vi "Withdrawal $50.vi"(8 "error in (no error)":errorcluster, 11 "ATM Controller in":refnum<class "ATM Controller.lvclass">) -> (0 "error out":errorcluster, 3 "ATM Controller out":refnum<class "ATM Controller.lvclass">)   [LabVIEW 2019, in "ATM Controller.lvlib" / "ATM Controller.lvclass"]
uses:
  ATM Controller.lvclass
  ATM Controller.lvclass/ATM Controller.ctl
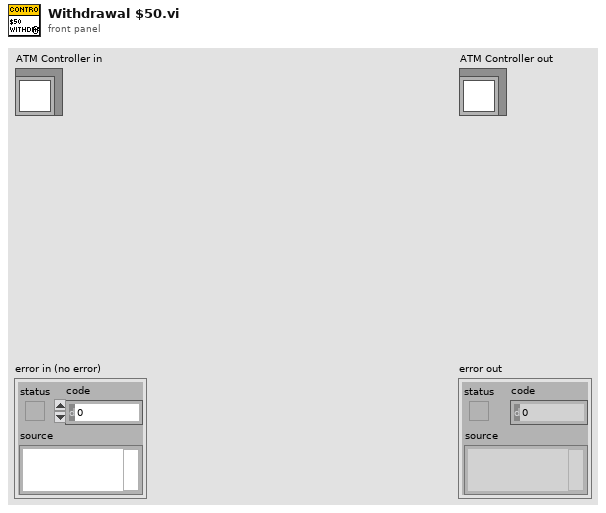
[diagram p1: front panel]
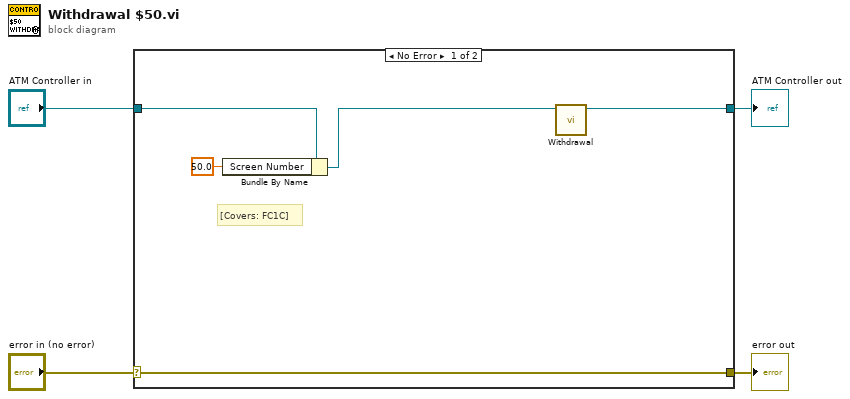
[diagram p0: block diagram]
diagram:
  n1 = case shown="No Error" "error in (no error)" {
    selector: "error in (no error)" -> [w9 w11]
    tunnel: [w9 w11] -> w3
    tunnel: [w8 w10] -> w1
    tunnel: "ATM Controller in" -> [w7 w10]
    frame No Error {
      # "[Covers: FC1C]"
      n2 = Bundle By Name(cluster=w7, "Screen Number"=50.0) -> (w5:refnum<class "ATM Controller.lvclass">)
      n3 = call "Withdrawal.vi"("ATM Controller in"=w5) -> ("ATM Controller out"=w8:refnum<class "ATM Controller.lvclass">)  [unwired: 9 in, 1 out]
    }
    frame Error {
    }
  }
  "error out" <- w3
  "ATM Controller out" <- w1
